vi "SimpleFunctionChose.vi"(6 "Method in":T1(ring), 9 "Parameters":dbl[](array[numeric]), 10 "x in":ext[](array[numeric]), 11 "Numeric":ext) -> (3 "x out":ext[](array[numeric]))   [LabVIEW 2016]
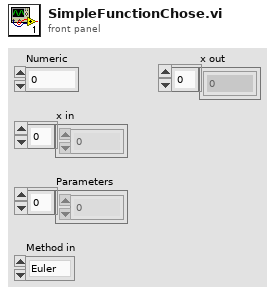
[diagram p1: front panel]
types:
  T1 = enum16{"Euler", "Cromer 1", "Cromer 2", "D1", "D2", "PD1", "PD2", "CD1", "CD2", "CD3", "CD4", "IMP", "LIMP", "IEuler", "SEMP", "SIMP", "EMP", "MEMP"}
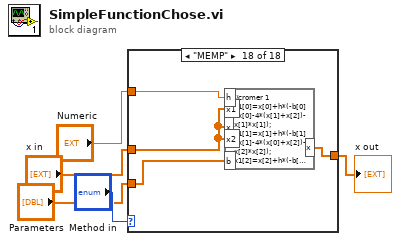
[diagram p0: block diagram]
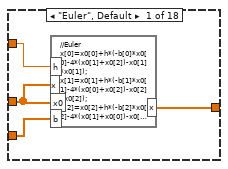
[diagram p2: hidden frame]
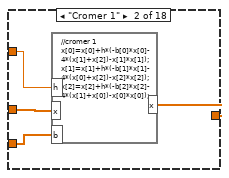
[diagram p3: hidden frame]
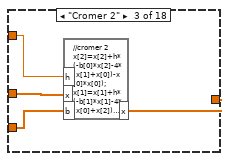
[diagram p4: hidden frame]
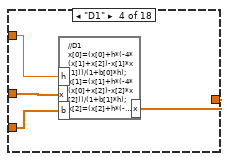
[diagram p5: hidden frame]
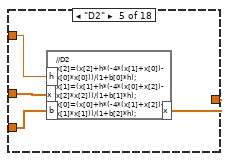
[diagram p6: hidden frame]
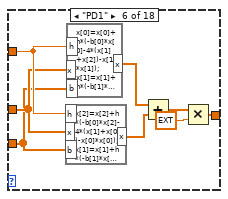
[diagram p7: hidden frame]
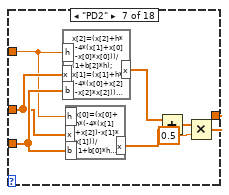
[diagram p8: hidden frame]
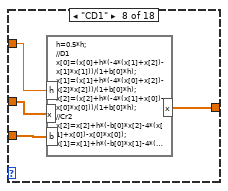
[diagram p9: hidden frame]
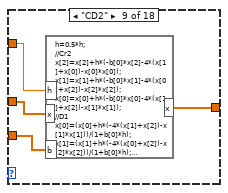
[diagram p10: hidden frame]
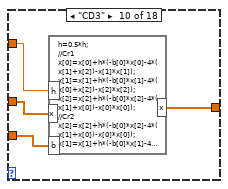
[diagram p11: hidden frame]
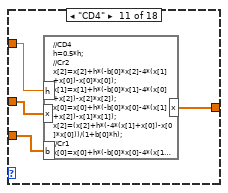
[diagram p12: hidden frame]
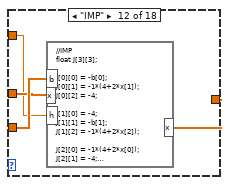
[diagram p13: hidden frame]
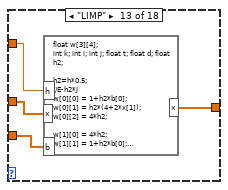
[diagram p14: hidden frame]
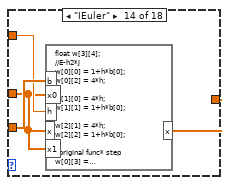
[diagram p15: hidden frame]
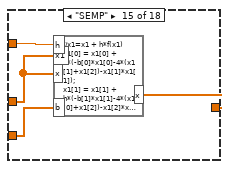
[diagram p16: hidden frame]
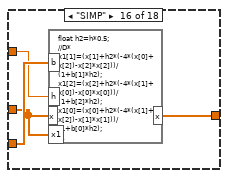
[diagram p17: hidden frame]
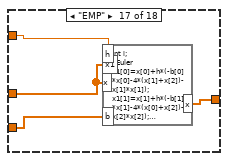
[diagram p18: hidden frame]
diagram:
  n1 = case shown="\"MEMP\"" "Method in" {
    tunnel: "Numeric" -> [w7 w13 w16 w20 w25 w28 w34 w44 w48 w53 w56 w58 w65 w68 w72 w75 w79 w83]
    tunnel: "Parameters" -> [w9 w11 w14 w18 w23 w26 w36 w42 w46 w51 w54 w60 w62 w69 w70 w76 w80 w84]
    tunnel: "x in" -> [w8 w12 w15 w19 w24 w27 w35 w43 w47 w52 w55 w59 w63 w67 w71 w74 w78 w85]
    tunnel: [w6 w10 w17 w21 w22 w29 w37 w45 w49 w50 w57 w61 w64 w66 w73 w77 w81 w82] -> w1
    frame "Euler", Default {
      n2 = formula code="//Euler\nx[0]=x0[0]+h*(-b[0]*x0[0]-4*(x0[1]+x0[2])-x0[1]*x0[1]);\nx[1]=x0[1]+h*(-b[1]*x0[1]-4*(x0[0]+x0[2])-x0[2]*x0[2]);\nx[2]=x0[2]+h*(-b[2]*x0[2]-4*(x0[1]+x0[0])-x0[0]*x0[0]);"("x"=w8, "x0"=w8, "b"=w9, "h"=w7) -> ("x"=w6:ext[])
    }
    frame "Cromer 1" {
      n3 = formula code="//cromer 1\nx[0]=x[0]+h*(-b[0]*x[0]-4*(x[1]+x[2])-x[1]*x[1]);\nx[1]=x[1]+h*(-b[1]*x[1]-4*(x[0]+x[2])-x[2]*x[2]);\nx[2]=x[2]+h*(-b[2]*x[2]-4*(x[1]+x[0])-x[0]*x[0]);"("x"=w12, "b"=w11, "h"=w13) -> ("x"=w10:ext[])
    }
    frame "Cromer 2" {
      n4 = formula code="//cromer 2\nx[2]=x[2]+h*(-b[0]*x[2]-4*(x[1]+x[0])-x[0]*x[0]);\nx[1]=x[1]+h*(-b[1]*x[1]-4*(x[0]+x[2])-x[2]*x[2]);\nx[0]=x[0]+h*(-b[2]*x[0]-4*(x[1]+x[2])-x[1]*x[1]);"("x"=w15, "b"=w14, "h"=w16) -> ("x"=w17:ext[])
    }
    frame "D1" {
      n5 = formula code="//D1\nx[0]=(x[0]+h*(-4*(x[1]+x[2])-x[1]*x[1]))/(1+b[0]*h);\nx[1]=(x[1]+h*(-4*(x[0]+x[2])-x[2]*x[2]))/(1+b[1]*h);\nx[2]=(x[2]+h*(-4*(x[1]+x[0])-x[0]*x[0]))/(1+b[2]*h);"("x"=w19, "b"=w18, "h"=w20) -> ("x"=w21:ext[])
    }
    frame "D2" {
      n6 = formula code="//D2\nx[2]=(x[2]+h*(-4*(x[1]+x[0])-x[0]*x[0]))/(1+b[0]*h);\nx[1]=(x[1]+h*(-4*(x[0]+x[2])-x[2]*x[2]))/(1+b[1]*h);\nx[0]=(x[0]+h*(-4*(x[1]+x[2])-x[1]*x[1]))/(1+b[2]*h);"("x"=w24, "b"=w23, "h"=w25) -> ("x"=w22:ext[])
    }
    frame "PD1" {
      n7 = formula code="x[2]=x[2]+h*(-b[0]*x[2]-4*(x[1]+x[0])-x[0]*x[0]);\nx[1]=x[1]+h*(-b[1]*x[1]-4*(x[0]+x[2])-x[2]*x[2]);\nx[0]=x[0]+h*(-b[2]*x[0]-4*(x[1]+x[2])-x[1]*x[1]);"("x"=w27, "b"=w26, "h"=w28) -> ("x"=w31:ext[])
      n8 = formula code="x[0]=x[0]+h*(-b[0]*x[0]-4*(x[1]+x[2])-x[1]*x[1]);\nx[1]=x[1]+h*(-b[1]*x[1]-4*(x[0]+x[2])-x[2]*x[2]);\nx[2]=x[2]+h*(-b[2]*x[2]-4*(x[1]+x[0])-x[0]*x[0]);"("x"=w27, "b"=w26, "h"=w28) -> ("x"=w30:ext[])
      n9 = Add(x=w30, y=w31) -> (x+y=w32:ext[])
      n10 = Multiply(x=w32, y=ext 0.5) -> (x*y=w29:ext[])
    }
    frame "PD2" {
      n11 = formula code="x[2]=(x[2]+h*(-4*(x[1]+x[0])-x[0]*x[0]))/(1+b[2]*h);\nx[1]=(x[1]+h*(-4*(x[0]+x[2])-x[2]*x[2]))/(1+b[1]*h);\nx[0]=(x[0]+h*(-4*(x[1]+x[2])-x[1]*x[1]))/(1+b[0]*h);"("x"=w35, "b"=w36, "h"=w34) -> ("x"=w41:ext[])
      n12 = formula code="x[0]=(x[0]+h*(-4*(x[1]+x[2])-x[1]*x[1]))/(1+b[0]*h);\nx[1]=(x[1]+h*(-4*(x[0]+x[2])-x[2]*x[2]))/(1+b[0]*h);\nx[2]=(x[2]+h*(-4*(x[1]+x[0])-x[0]*x[0]))/(1+b[0]*h);"("x"=w35, "b"=w36, "h"=w34) -> ("x"=w40:ext[])
      n13 = Add(x=w41, y=w40) -> (x+y=w39:ext[])
      n14 = Multiply(x=w39, y=0.5) -> (x*y=w37:ext[])
    }
    frame "CD1" {
      n15 = formula code="h=0.5*h;\n//D1\nx[0]=(x[0]+h*(-4*(x[1]+x[2])-x[1]*x[1]))/(1+b[0]*h);\nx[1]=(x[1]+h*(-4*(x[0]+x[2])-x[2]*x[2]))/(1+b[0]*h);\nx[2]=(x[2]+h*(-4*(x[1]+x[0])-x[0]*x[0]))/(1+b[0]*h);\n//Cr2\nx[2]=x[2]+h*(-b[0]*x[2]-4*(x[1]+x[0])-x[0]*x[0]);\nx[1]=x[1]+h*(-b[0]*x[1]-4*(x[0]+x[2])-x[2]*x[2]);\nx[0]=x[0]+h*(-b[0]*x[0]-4*(x[1]+x[2])-x[1]*x[1]);"("x"=w43, "b"=w42, "h"=w44) -> ("x"=w45:ext[])
    }
    frame "CD2" {
      n16 = formula code="h=0.5*h;\n//Cr2\nx[2]=x[2]+h*(-b[0]*x[2]-4*(x[1]+x[0])-x[0]*x[0]);\nx[1]=x[1]+h*(-b[0]*x[1]-4*(x[0]+x[2])-x[2]*x[2]);\nx[0]=x[0]+h*(-b[0]*x[0]-4*(x[1]+x[2])-x[1]*x[1]);\n//D1\nx[0]=(x[0]+h*(-4*(x[1]+x[2])-x[1]*x[1]))/(1+b[0]*h);\nx[1]=(x[1]+h*(-4*(x[0]+x[2])-x[2]*x[2]))/(1+b[0]*h);\nx[2]=(x[2]+h*(-4*(x[1]+x[0])-x[0]*x[0]))/(1+b[0]*h);"("x"=w47, "b"=w46, "h"=w48) -> ("x"=w49:ext[])
    }
    frame "CD3" {
      n17 = formula code="h=0.5*h;\n//Cr1\nx[0]=x[0]+h*(-b[0]*x[0]-4*(x[1]+x[2])-x[1]*x[1]);\nx[1]=x[1]+h*(-b[0]*x[1]-4*(x[0]+x[2])-x[2]*x[2]);\nx[2]=x[2]+h*(-b[0]*x[2]-4*(x[1]+x[0])-x[0]*x[0]);\n//Cr2\nx[2]=x[2]+h*(-b[0]*x[2]-4*(x[1]+x[0])-x[0]*x[0]);\nx[1]=x[1]+h*(-b[0]*x[1]-4*(x[0]+x[2])-x[2]*x[2]);\nx[0]=x[0]+h*(-b[0]*x[0]-4*(x[1]+x[2])-x[1]*x[1]);"("x"=w52, "b"=w51, "h"=w53) -> ("x"=w50:ext[])
    }
    frame "CD4" {
      n18 = formula code="//CD4\nh=0.5*h;\n//Cr2\nx[2]=x[2]+h*(-b[0]*x[2]-4*(x[1]+x[0])-x[0]*x[0]);\nx[1]=x[1]+h*(-b[0]*x[1]-4*(x[0]+x[2])-x[2]*x[2]);\nx[0]=x[0]+h*(-b[0]*x[0]-4*(x[1]+x[2])-x[1]*x[1]);\nx[2]=(x[2]+h*(-4*(x[1]+x[0])-x[0]*x[0]))/(1+b[0]*h);\n//Cr1\nx[0]=x[0]+h*(-b[0]*x[0]-4*(x[1]+x[2])-x[1]*x[1]);\nx[1]=x[1]+h*(-b[0]*x[1]-4*(x[0]+x[2])-x[2]*x[2]);\nx[2]=x[2]+h*(-b[0]*x[2]-4*(x[1]+x[0])-x[0]*x[0]);"("x"=w55, "b"=w54, "h"=w56) -> ("x"=w57:ext[])
    }
    frame "IMP" {
      n19 = formula code="//IMP\nfloat J[3][3];\n\nJ[0][0] = -b[0]; \nJ[0][1] = -1*(4+2*x[1]); \nJ[0][2] = -4; \n\nJ[1][0] = -4; \nJ[1][1] = -b[1];\nJ[1][2] = -1*(4+2*x[2]);\n\nJ[2][0] = -1*(4+2*x[0]); \nJ[2][1] = -4;\nJ[2][2] = -b[2];\n\n\nfloat w[3][4], Z[3], a[3], Zn[3], dz;\nfloat tol;\nint k; int i; int j; float t; float d;\ntol = 1e-14;\nint nnewtmax = 3, nnewt;\ndz = 2e-13;\nnnewt = 0;\n\nZ[0] = x[0]; Z[1] = x[1]; Z[2] = x[2];\nwhile ( (dz > tol) && (nnewt < nnewtmax)){\n\tfor(i=0;i<3;i++)\n\t{\n\t\tfor(j=0;j<3;j++)\n\t\t{\n\t\t\tif (i==j)\n\t\t\tw[i][j]=1 - 0.5*h*J[i][j];\n\t\t\telse\n\t\t\tw[i][j]= - 0.5*h*J[i][j];\n\t\t}\n\t}\n\n\n\n\ta[0] = 0.5*(x[0] + Z[0]);\n\ta[1] = 0.5*(x[1] + Z[1]);\n\ta[2] = 0.5*(x[2] + Z[2]);\n\t\n\tw[0][3]= -Z[0]+x[0]+h*(-b[0]*a[0]-4*(a[1]+a[2])-a[1]*a[1]);\n\tw[1][3]= -Z[1]+x[1]+h*(-b[1]*a[1]-4*(a[0]+a[2])-a[2]*a[2]);\n\tw[2][3]= -Z[2]+x[2]+h*(-b[2]*a[2]-4*(a[1]+a[0])-a[0]*a[0]);\n\t\n\t\n\tfor(k = 0; k <= 1; k++){\n\t\tint l = k;\n\t\n\t\tfor( i = k+1; i<= 2; i++){\n\t\t\tif( abs(w[i][k]) > abs(w[l][k]) ){\n\t\t\tl = i;\n\t\t\t}\n\t\t}\n\t\tif (l != k){\n\t\t\tfor( j = 0; j <= 3; j++){\n\t\t\t\tif ((j == 0) || (j >= k)){\n\t\t\t\t\tt = w[k][j];\n\t\t\t\t\tw[k][j] = w[l][j];\n\t\t\t\t\tw[l][j] = t;\n\t\t\t\t}\n\t\t\t}\n\t\t}\t\n\n\t\td = 1.0 / w[k][k];\n\t\tfor( i=(k+1); i <=(2); i++){\n\t\t\tif (w[i][k] == 0){\n\t\t\t\tcontinue;\n\t\t\t}\n\t\t\tt = w[i][k] * d;\n\t\t\tfor ( j = k; j <= (3); j++) {\n\t\t\t\tif (w[k][j] != 0){\n\t\t\t\t\tw[i][j] = w[i][j] - t * w[k][j];\n\t\t\t\t}\n\t\t\t}\n\t\t}\n\t}\n\tfor( i=(3); i >= 2; i--){\n\t\tfor( j=1; j <= i-1; j++){\n\t\t\tt = w[i - j - 1][i - 1]/w[ i -1][i - 1];\n\t\t\tw[i-j - 1][ 3] = w[i-j -1][3] - t*w[i - 1][ 3];\n\t\t}\n\t\tw[i-1][ 3] = w[i - 1][3]/w[ i -1][i - 1];\n\t}\n\tw[0][3] = w[0][3]/w[0][0];\n\tZn[0] = Z[0]+ w[0][3];\n\tZn[1] = Z[1]+ w[1][3];\n\tZn[2] = Z[2]+ w[2][3];\n\t\n\tdz = ( (Zn[0] - Z[0])**2 + (Zn[1] - Z[1])**2 + (Zn[2] - Z[2])**2 )**0.5;\n\tZ[0] = Zn[0];\n\tZ[1] = Zn[1];\n\tZ[2] = Zn[2];\n\n\tnnewt ++;\n}\n\nx[0] = Zn[0];\nx[1] = Zn[1];\nx[2] = Zn[2];"("x"=w59, "h"=w58, "b"=w60) -> ("x"=w61:ext[])
    }
    frame "LIMP" {
      n20 = formula code="float w[3][4];\nint k; int i; int j; float t; float d; float h2;\n\nh2=h*0.5;\n//E-h2*J\nw[0][0] = 1+h2*b[0];\nw[0][1] = h2*(4+2*x[1]);\nw[0][2] = 4*h2;\n\nw[1][0] = 4*h2;\nw[1][1] = 1+h2*b[0];\nw[1][2] = h2*(4+2*x[2]);\n\nw[2][0] = h2*(4+2*x[0]);\nw[2][1] = 4*h2;\nw[2][2] = 1+h2*b[0];\n\n//original func* step\nw[0][3] = h*(-b[0]*x[0]-4*(x[1]+x[2])-x[1]*x[1]);\nw[1][3] = h*(-b[0]*x[1]-4*(x[0]+x[2])-x[2]*x[2]);\nw[2][3] = h*(-b[0]*x[2]-4*(x[1]+x[0])-x[0]*x[0]);\n\n\nint HEIGHT = 3;\nint  WIDTH = 4;\nfor(k = 0; k <= HEIGHT-2; k++){\n\nint\tl = k;\n\nfor( i = k+1;  i<= HEIGHT-1; i++){\n\t\t\tif( abs(w[i][k]) > abs(w[l][k]) ){\n\t\t\t\tl = i;\n    }\n   }\n\t\tif (l != k){\n\t\t\tfor( j = 0; j <= WIDTH-1; j++){\n\t\t\t\tif ((j == 0) || (j >= k)){\n\t\t\t\t\tt = w[k][j];\n\t\t\t\t\tw[k][j] = w[l][j];\n\t\t\t\t\tw[l][j] = t;\n                }\n            }\n        }\n\n\t\td = 1.0 / w[k][k];\n\t\tfor( i=(k+1); i <=(HEIGHT-1); i++){\n\t\t\tif (w[i][k] == 0){\n                continue;\n            }\n\t\t\tt = w[i][k] * d;\n\t\t\tfor ( j = k; j <= (WIDTH-1); j++) {\n\t\t\t\tif (w[k][j] != 0){\n\t\t\t\t\tw[i][j] = w[i][j] - t * w[k][j];\n                }\n            }\n        }\n    }\n    \n\t\n    for( i=(HEIGHT); i >= 2; i--){ \n        for( j=1; j <= i-1; j++){\n            t = w[i - j - 1][i - 1]/w[ i -1][i - 1];\n            w[i-j - 1][ WIDTH- 1] = w[i-j -1][ WIDTH -1] - t*w[i - 1][ WIDTH -1];\n        }\n        w[i-1][ WIDTH-1] = w[i - 1][ WIDTH - 1]/w[ i -1][i - 1];\n    }\n    w[0][ WIDTH - 1] = w[0][ WIDTH -1]/w[0][0];\n\n    \n    x[0] =x[0]+ w[0][WIDTH - 1];\n    x[1] = x[1]+w[1][WIDTH - 1];\n    x[2] = x[2]+w[2][WIDTH - 1];"("x"=w63, "b"=w62, "h"=w65) -> ("x"=w64:ext[])
    }
    frame "IEuler" {
      n21 = formula code="float w[3][4];\n//E-h2*J\nw[0][0] = 1+h*b[0];\nw[0][2] = 4*h;\n\nw[1][0] = 4*h;\nw[1][1] = 1+h*b[0];\n\nw[2][1] = 4*h;\nw[2][2] = 1+h*b[0];\n\n//original func* step\nw[0][3] = h*(-b[0]*x[0]-4*(x[1]+x[2])-x[1]*x[1]);\nw[1][3] = h*(-b[0]*x[1]-4*(x[0]+x[2])-x[2]*x[2]);\nw[2][3] = h*(-b[0]*x[2]-4*(x[1]+x[0])-x[0]*x[0]);\n\nfloat tol = 1e-12;\nfloat dx = 2*tol;\n\nint nmax = 10;\nint n = 0;\n//цикл по Ньютонам\nwhile ((dx > tol)&&(n < nmax)){\n\n\tw[0][1] = h*(4+2*x[1]);\n\tw[1][2] = h*(4+2*x[2]);\n\tw[2][0] = h*(4+2*x[0]);\n\n\tw[0][3] = x0[0] - x1[0] + h*(-b[0]*x[0]-4*(x[1]+x[2])-x[1]*x[1]);\n\tw[1][3] = x0[1] - x1[1] + h*(-b[0]*x[1]-4*(x[0]+x[2])-x[2]*x[2]);\n\tw[2][3] = x0[2] - x1[2] + h*(-b[0]*x[2]-4*(x[1]+x[0])-x[0]*x[0]);\n\n\tint HEIGHT = 3;\n\tint  WIDTH = 4;\n\tint k; int i; int j; float t; float d;\n\n\tfor(k = 0; k <= HEIGHT-2; k++){\n\t\tint\tl = k;\n\t\tfor( i = k+1;  i<= HEIGHT-1; i++){\n\t\t\t\t\tif( abs(w[i][k]) > abs(w[l][k]) ){\n\t\t\t\t\t\tl = i;\n\t\t\t}\n\t   }\n\t\t\tif (l != k){\n\t\t\t\tfor( j = 0; j <= WIDTH-1; j++){\n\t\t\t\t\tif ((j == 0) || (j >= k)){\n\t\t\t\t\t\tt = w[k][j];\n\t\t\t\t\t\tw[k][j] = w[l][j];\n\t\t\t\t\t\tw[l][j] = t;\n\t\t\t\t\t}\n\t\t\t\t}\n\t\t\t}\n\t\t\t\n\t\t\td = 1.0 / w[k][k];\n\t\t\tfor( i=(k+1); i <=(HEIGHT-1); i++){\n\t\t\t\tif (w[i][k] == 0){\n\t\t\t\t\tcontinue;\n\t\t\t\t}\n\t\t\t\tt = w[i][k] * d;\n\t\t\t\tfor ( j = k; j <= (WIDTH-1); j++) {\n\t\t\t\t\tif (w[k][j] != 0){\n\t\t\t\t\t\tw[i][j] = w[i][j] - t * w[k][j];\n\t\t\t\t\t}\n\t\t\t\t}\n\t\t\t}\n\t\t}\n\n\t\tfor( i=(HEIGHT); i >= 2; i--){ \n\t\t\tfor( j=1; j <= i-1; j++){\n\t\t\t\tt = w[i - j - 1][i - 1]/w[ i -1][i - 1];\n\t\t\t\tw[i-j - 1][ WIDTH- 1] = w[i-j -1][ WIDTH -1] - t*w[i - 1][ WIDTH -1];\n\t\t\t}\n\t\t\tw[i-1][ WIDTH-1] = w[i - 1][ WIDTH - 1]/w[ i -1][i - 1];\n\t\t}\n\t\tw[0][ WIDTH - 1] = w[0][ WIDTH -1]/w[0][0];\n\n\t\t\n\t\tx1[0] =x[0]+ w[0][WIDTH - 1];\n\t\tx1[1] = x[1]+w[1][WIDTH - 1];\n\t\tx1[2] = x[2]+w[2][WIDTH - 1];\n\n\tdx = sqrt((x1[0] - x[0])**2 + (x1[1] - x[1])**2 + (x1[2] - x[2])**2);\n\tn++;\n\n\tx[0] = x1[0]; x[1] = x1[1]; x[2] = x1[2];\n\n}"("x"=w67, "h"=w68, "x1"=w67, "b"=w69, "x0"=w67) -> ("x"=w66:ext[])
    }
    frame "SEMP" {
      n22 = formula code="//x1=x1 + h*f(x1)\nx1[0] = x1[0] + h*(-b[0]*x1[0]-4*(x1[1]+x1[2])-x1[1]*x1[1]); \nx1[1] = x1[1] + h*(-b[1]*x1[1]-4*(x1[0]+x1[2])-x1[2]*x1[2]); \nx1[2] = x1[2] + h*(-b[2]*x1[2]-4*(x1[1]+x1[0])-x1[0]*x1[0]);\n\n\n//x+h*f(x1)\nx[0] = x[0] + h*(-b[0]*x1[0]-4*(x1[1]+x1[2])-x1[1]*x1[1]); \nx[1] = x[1] + h*(-b[1]*x1[1]-4*(x1[0]+x1[2])-x1[2]*x1[2]); \nx[2] = x[2] + h*(-b[2]*x1[2]-4*(x1[1]+x1[0])-x1[0]*x1[0]);"("x"=w71, "x1"=w71, "h"=w72, "b"=w70) -> ("x"=w73:ext[])
    }
    frame "SIMP" {
      n23 = formula code="float h2=h*0.5;\n//D*\nx1[1]=(x[1]+h2*(-4*(x[0]+x[2])-x[2]*x[2]))/(1+b[1]*h2);\nx1[2]=(x[2]+h2*(-4*(x[1]+x[0])-x[0]*x[0]))/(1+b[2]*h2);\nx1[0]=(x[0]+h2*(-4*(x[1]+x[2])-x[1]*x[1]))/(1+b[0]*h2);\n\n\n//??\nx[0]=x[0]+h*(-b[0]*x1[0]-4*(x1[1]+x1[2])-x1[1]*x1[1]);\nx[1]=x[1]+h*(-b[1]*x1[1]-4*(x1[0]+x1[2])-x1[2]*x1[2]);\nx[2]=x[2]+h*(-b[2]*x1[2]-4*(x1[1]+x1[0])-x1[0]*x1[0]);"("x"=w74, "h"=w75, "x1"=w74, "b"=w76) -> ("x"=w77:ext[])
    }
    frame "EMP" {
      n24 = formula code="int i;\n//Euler\nx1[0]=x[0]+h*(-b[0]*x[0]-4*(x[1]+x[2])-x[1]*x[1]);\nx1[1]=x[1]+h*(-b[1]*x[1]-4*(x[0]+x[2])-x[2]*x[2]);\nx1[2]=x[2]+h*(-b[2]*x[2]-4*(x[1]+x[0])-x[0]*x[0]);\n\n//EEuler\nx[0]=x[0]+h*(-b[0]*x1[0]-4*(x1[1]+x1[2])-x1[1]*x1[1]);\nx[1]=x[1]+h*(-b[1]*x1[1]-4*(x1[0]+x1[2])-x1[2]*x1[2]);\nx[2]=x[2]+h*(-b[2]*x1[2]-4*(x1[1]+x1[0])-x1[0]*x1[0]);"("x"=w78, "x1"=w78, "h"=w79, "b"=w80) -> ("x"=w81:ext[])
    }
    frame "MEMP" {
      n25 = formula code="//cromer 1\nx1[0]=x[0]+h*(-b[0]*x[0]-4*(x[1]+x[2])-x[1]*x[1]);\nx1[1]=x[1]+h*(-b[1]*x[1]-4*(x[0]+x[2])-x[2]*x[2]);\nx1[2]=x[2]+h*(-b[2]*x[2]-4*(x[1]+x[0])-x[0]*x[0]);\nh=2*h;\n\n//EEuler\nx2[0]=x[0]+h*(-b[0]*x1[0]-4*(x1[1]+x1[2])-x1[1]*x1[1]);\nx2[1]=x[1]+h*(-b[1]*x1[1]-4*(x1[0]+x1[2])-x1[2]*x1[2]);\nx2[2]=x[2]+h*(-b[2]*x1[2]-4*(x1[1]+x1[0])-x1[0]*x1[0]);\n\nx[0]=x1[0];\nx[1]=x1[1];\nx[2]=x1[2];\nx1[0]=x2[0];\nx1[1]=x2[1];\nx1[2]=x2[2];\nh=h*0.5;\nx[0]=(x[0]+x1[0]+h*(-b[0]*x1[0]-4*(x1[1]+x1[2])-x1[1]*x1[1]))/2;\nx[1]=(x[1]+x1[1]+h*(-b[1]*x1[1]-4*(x1[0]+x1[2])-x1[2]*x1[2]))/2;\nx[2]=(x[2]+x1[2]+h*(-b[2]*x1[2]-4*(x1[1]+x1[0])-x1[0]*x1[0]))/2;"("x"=w85, "x1"=w85, "h"=w83, "b"=w84, "x2"=w85) -> ("x"=w82:ext[])
    }
  }
  "x out" <- w1
